vi "3.2.vi"() -> ()   [LabVIEW 2017]
panel:
  in  "功能选择":enum16{"相加", "相乘", "相减", "相除"}(ring)
  out "result":dbl
  in  "B":dbl
  in  "A":dbl
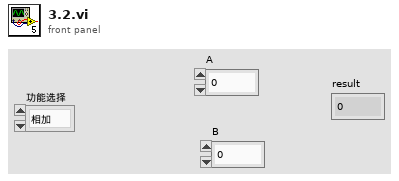
[diagram p1: front panel]
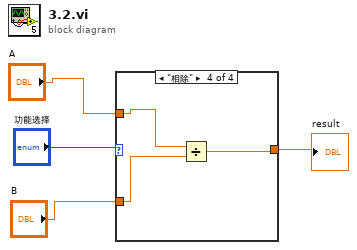
[diagram p0: block diagram]
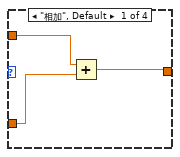
[diagram p2: hidden frame]
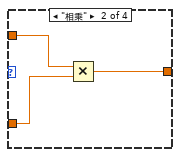
[diagram p3: hidden frame]
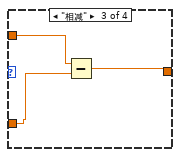
[diagram p4: hidden frame]
diagram:
  n1 = case shown="\"相除\"" "功能选择" {
    tunnel: "A" -> [w7 w10 w13 w15]
    tunnel: "B" -> [w6 w9 w12 w14]
    tunnel: [w5 w8 w11 w16] -> w1
    frame "相加", Default {
      n2 = Add(x=w7, y=w6) -> (x+y=w5:dbl)
    }
    frame "相乘" {
      n3 = Multiply(x=w10, y=w9) -> (x*y=w8:dbl)
    }
    frame "相减" {
      n4 = Subtract(x=w13, y=w12) -> (x-y=w11:dbl)
    }
    frame "相除" {
      n5 = Divide(x=w15, y=w14) -> (x/y=w16:dbl)
    }
  }
  "result" <- w1
